vi "SET Enqueuers Array 2 Dispatch Message.vi"(8 "error in (no error)":errorcluster, 10 "Enqueuers Array":refnum<class "Message Enqueuer.lvclass">[](array[class]), 11 "Child_1_Class in":refnum<class "GUI_Class.lvclass">) -> (0 "error out":errorcluster, 3 "Child_1_Class out":refnum<class "GUI_Class.lvclass">)   [LabVIEW 2023, in "GUI_Actor.lvlib" / "GUI_Class.lvclass"]
uses:
  GUI_Class.lvclass
  <vilib>/ActorFramework/Message Enqueuer/Message Enqueuer.lvclass
  GUI - Ctrl - Trigger Event Cluster.ctl
  Usr Ev/GUI - Ctrl - Enum - Events.ctl
  GUI_Class.lvclass/GUI_Class.ctl
panel:
  out "Child Trigger Event Cluster":T1
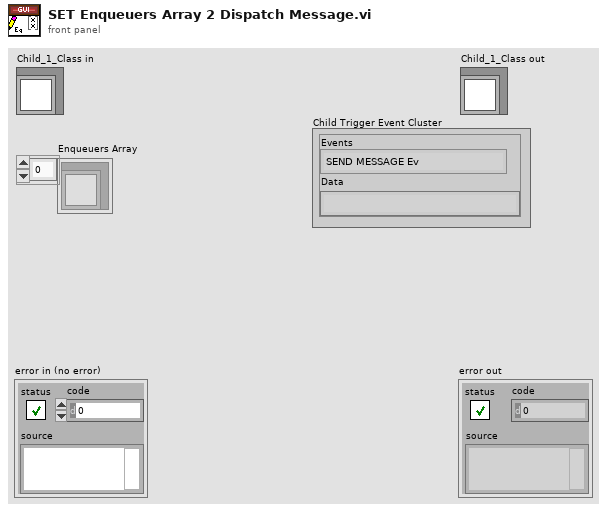
[diagram p1: front panel]
types:
  T1 = typedef "GUI_Actor.lvlib/GUI_Class.lvclass/GUI - Ctrl - Trigger Event Cluster.ctl" = cluster{"Events":T2, "Data":string}
  T2 = typedef "GUI_Actor.lvlib/GUI_Class.lvclass/GUI - Ctrl - Enum - Events.ctl" = enum16{"SEND MESSAGE Ev", "STOP_ACTOR Ev", "INIT_ACTOR Ev", "START Ev", "STOP Ev", "GET Ev", "SET Ev", "ERROR_HANDLER Ev", "RESET Ev", "T2 Ev", "T3 Ev", "T4 Ev"}
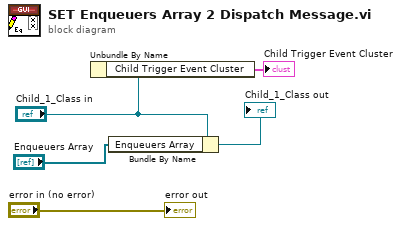
[diagram p0: block diagram]
diagram:
  n1 = Unbundle By Name("Child_1_Class in") -> ("Child Trigger Event Cluster"=→"Child Trigger Event Cluster":T1)
  n2 = Bundle By Name(cluster="Child_1_Class in", "Enqueuers Array"="Enqueuers Array") -> (→"Child_1_Class out":refnum<class "GUI_Class.lvclass">)
  "error out" <- "error in (no error)"
